vi "Encode String.vi"(10 "String":string, 11 "URI-Component":refnum<class "URI-Component.lvclass">) -> (2 "Encoded String":string)   [LabVIEW 2013, in "openURI.lvlib" / "URI-Component.lvclass"]
uses:
  URI-Component.lvclass
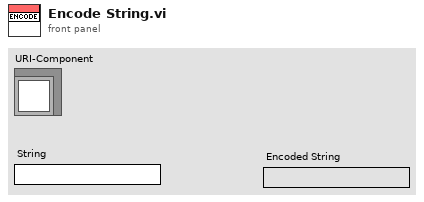
[diagram p1: front panel]
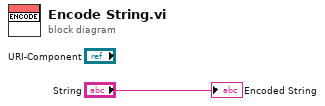
[diagram p0: block diagram]
diagram:
  "Encoded String" <- "String"
